vi "fitGaussian2DMarginals.vi"(1 "Image In":dbl[][](array[numeric])) -> (0 "parameters out":cluster{"X":dbl[], "Y":dbl[]} {"X" format="%#_6f"; "Y" format="%#_6f"})   [LabVIEW 2017]
panel:
  out "Waveform Graph 2":dbl[](graph)
  out "Waveform Graph":dbl[][](graph)
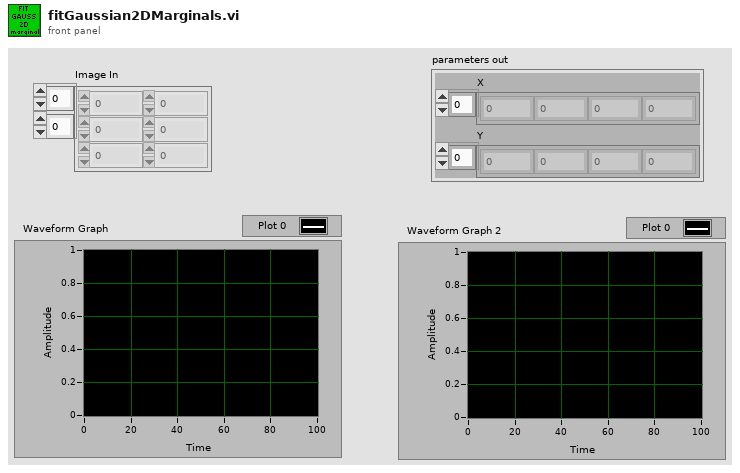
[diagram p1: front panel]
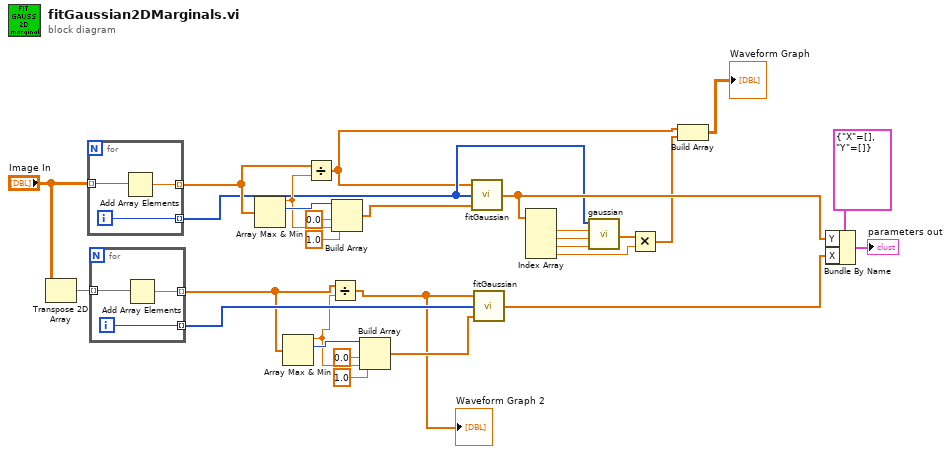
[diagram p0: block diagram]
diagram:
  n1 = Transpose 2D Array(2D array="Image In") -> (transposed array=w28:dbl[][])
  n2 = for {
    tunnel: "Image In" -> [w32] mode=indexing
    tunnel: [w31] -> w19 mode=indexing
    tunnel: [w30] -> w9 mode=indexing
    i -> [w30]
    n3 = Add Array Elements(numeric array=w32) -> (sum=w31:dbl)
  }
  n4 = for {
    tunnel: w28 -> [w35] mode=indexing
    tunnel: [w34] -> w13 mode=indexing
    tunnel: [w33] -> w27 mode=indexing
    i -> [w33]
    n5 = Add Array Elements(numeric array=w35) -> (sum=w34:dbl)
  }
  n6 = Array Max & Min(array=w19) -> (max value=w18:dbl, max index (indices)=w23:i32)  [unwired: 2 out]
  n7 = Array Max & Min(array=w13) -> (max value=w12:dbl, max index (indices)=w14:i32)  [unwired: 2 out]
  n8 = Divide(x=w19, y=w18) -> (x/y=w3:dbl[])
  n9 = Divide(x=w13, y=w12) -> (x/y=w11:dbl[])
  "Waveform Graph 2" <- w11
  n10 = Build Array(w23, 1.0 ("element"), 0.0 ("element"), w18) -> (w20:dbl[])
  n11 = Build Array(w14, 1.0 ("element"), 0.0 ("element"), w12) -> (w15:dbl[])
  n12 = call "fitGaussian.vi"("initial parameters"=w20, "X"=w9, "Y"=w3) -> ("x0,sigma,bg,amplitude"=w10:dbl[])
  n13 = call "fitGaussian.vi"("initial parameters"=w15, "X"=w27, "Y"=w11) -> ("x0,sigma,bg,amplitude"=w24:dbl[])
  n14 = Index Array(array=w10) -> (element #1=w8:dbl, element #2=w7:dbl, element #3=w6:dbl, element #4=w4:dbl)  [unwired: 4 in]
  n15 = call "gaussian.vi"("bg"=w6, "sigma"=w7, "x0"=w8, "X"=w9) -> ("Y"=w5:dbl[])
  n16 = Multiply(x=w5, y=w4) -> (x*y=w2:dbl[])
  n17 = Build Array(w3, w2) -> (→"Waveform Graph":dbl[][])
  n18 = Bundle By Name(cluster=cluster{"X":dbl[], "Y":dbl[]} {"X"=[], "Y"=[]} ("input cluster"), "Y"=w10, "X"=w24) -> (→"parameters out":cluster{"X":dbl[], "Y":dbl[]})
